vi "XmlLogger_Init.vi"(0 "object in":refnum<class "XmlLogger.lvclass">, 2 "LogString":refnum<vi>, 5 "error in (no error)":errorcluster) -> (14 "object out":refnum<class "XmlLogger.lvclass">, 19 "error out":errorcluster)   [LabVIEW 2014, in "XmlLogger.lvclass"]
uses:
  XmlLogger.lvclass
  XmlLogger.lvclass/XmlLogger.ctl
  Logger_class/Logger.lvclass
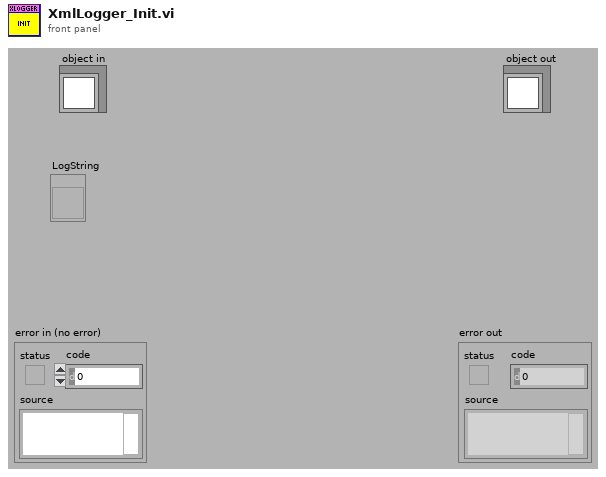
[diagram p1: front panel]
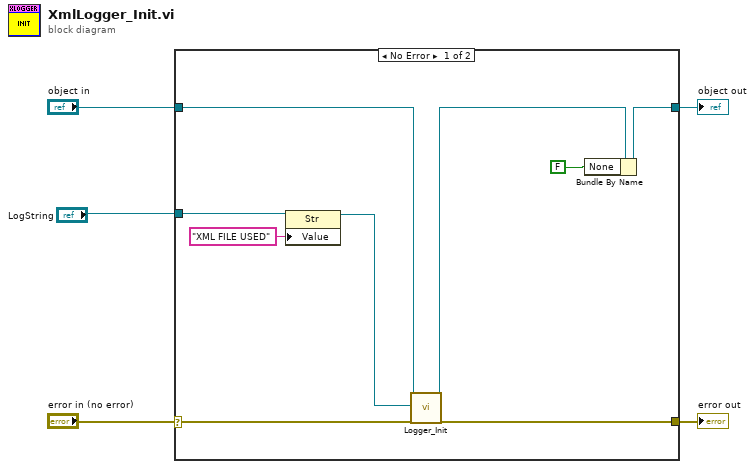
[diagram p0: block diagram]
diagram:
  n1 = case shown="No Error" "error in (no error)" {
    selector: "error in (no error)" -> [w12 w15]
    tunnel: [w14 w16] -> w5
    tunnel: "object in" -> [w10 w16]
    tunnel: [w11 w15] -> w2
    tunnel: "LogString" -> [w8 _]
    frame No Error {
      n2 = property class="Str"(reference=w8, "Value"="XML FILE USED") -> (reference out=w6:refnum<vi>)  [unwired: 1 in, 1 out]
      n3 = call "Logger_Init.vi"("object in"=w10, "LogString"=w6, "error in (no error)"=w12) -> ("object out"=w9:refnum<class "XmlLogger.lvclass">, "error out"=w11:errorcluster)  [unwired: 15 in]
      n4 = Bundle By Name(cluster=w9, "None"=FALSE) -> (w14:refnum<class "XmlLogger.lvclass">)
    }
    frame Error {
    }
  }
  "object out" <- w5
  "error out" <- w2
